vi "cleanRAWobj.vi"(8 "error in (no error)":errorcluster, 11 "raw dxf obj in":string) -> (0 "error out":errorcluster, 3 "dxfObject":T1, 5 "complete obj as 2Darray out":string[][](array[string]))   [LabVIEW 2016, in "Dxf.lvlib"]
uses:
  Dxf.lvlib
  typeDefs/singleDXFobject.ctl
  typeDefs/singleDXFvar.ctl
  <vilib>/Utility/error.llb/whitespace.ctl
  dxf typedef.lvlib
panel:
  out "raw obj cleaned":string
  # "Connector Pane"
  # "Locals"
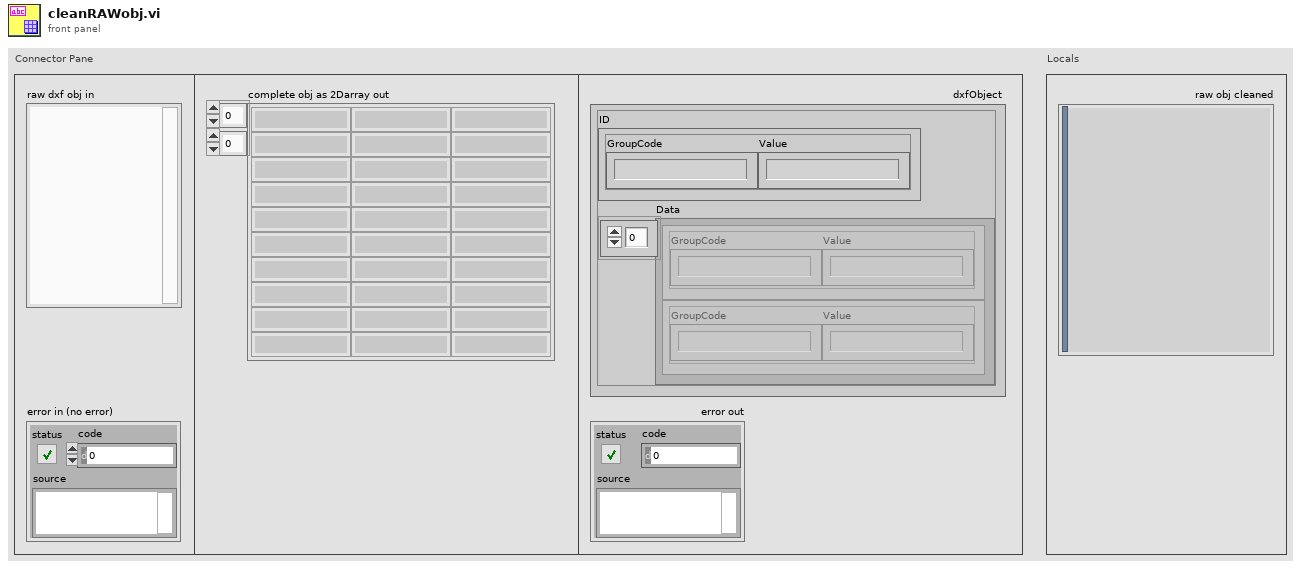
[diagram p1: front panel]
types:
  T1 = typedef "dxf typedef.lvlib/singleDXFobject.ctl" = cluster{"ID":T2, "Data":T2[]}
  T2 = typedef "dxf typedef.lvlib/singleDXFvar.ctl" = cluster{"GroupCode":string, "Value":string}
  T3 = typedef "whitespace.ctl" = u16
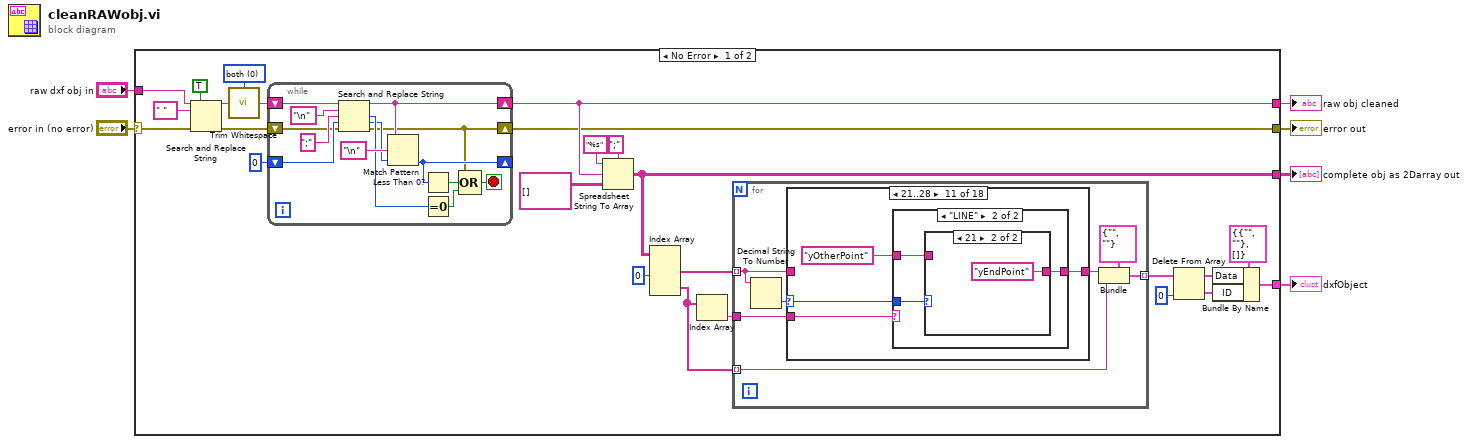
[diagram p0: block diagram]
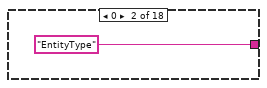
[diagram p3: hidden frame]
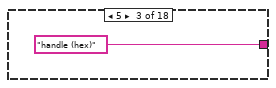
[diagram p4: hidden frame]
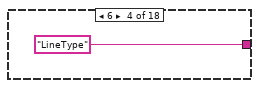
[diagram p5: hidden frame]
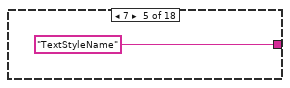
[diagram p6: hidden frame]
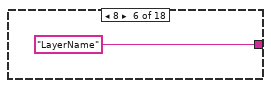
[diagram p7: hidden frame]
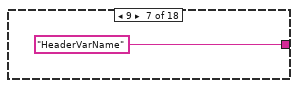
[diagram p8: hidden frame]
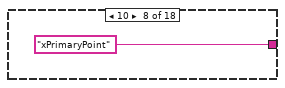
[diagram p9: hidden frame]
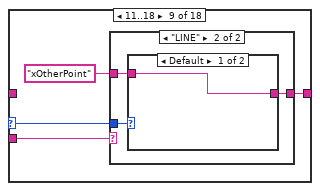
[diagram p10: hidden frame]
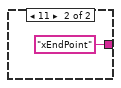
[diagram p12: hidden frame]
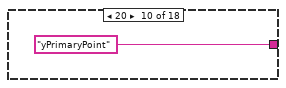
[diagram p13: hidden frame]
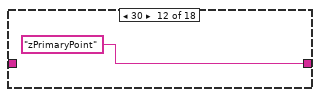
[diagram p16: hidden frame]
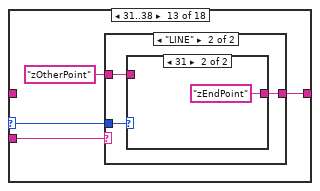
[diagram p17: hidden frame]
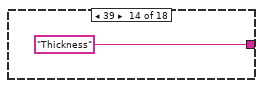
[diagram p20: hidden frame]
diagram:
  n1 = case shown="No Error" "error in (no error)" {
    selector: "error in (no error)" -> [w21 w122]
    tunnel: [w28 _] -> w6
    tunnel: [w17 _] -> w5
    tunnel: [w19 w122] -> w3
    tunnel: "raw dxf obj in" -> [w18 _]
    tunnel: [w12 _] -> w1
    frame No Error {
      w22 = T3 0 items=["both", "start of string", "end of string"] ("location (both)")
      n2 = Search and Replace String(replace all?=TRUE ("replace all? (F)"), input string=w18, search string=" ", error in=w21) -> (result string=w26:string, error out=w20:errorcluster)  [unwired: 4 in, 2 out]
      n3 = call <vilib>:"Trim Whitespace.vi"("string"=w26, "location (both)"=w22) -> ("trimmed string"=w23:string)
      n4 = while {
        shift-right: [w115] -> w28
        shift-left: w23 -> [w120]
        shift-right: [w111] -> _
        shift-left: 0 ("offset past match") -> [w116]
        shift-right: [w108] -> w19
        shift-left: w20 -> [w109]
        stop <- w114 stop-if-true
        n5 = Search and Replace String(input string=w120, search string="\n", replace string=";" ("replace string (\"\")"), offset=w116, error in=w109) -> (result string=w115:string, number of replacements=w113:i32, offset past replacement=w112:i32, error out=w108:errorcluster)  [unwired: 3 in]
        n6 = Match Pattern(string=w115, regular expression="\n" ("search string"), offset (0)=w112) -> (offset past match=w111:i32)  [unwired: 3 out]
        n7 = Less Than 0?(x=w111) -> (x < 0?=w110:bool)
        n8 = Equal To 0?(x=w113) -> (x = 0?=w121:bool)
        n9 = Compound Arithmetic op=OR(w108, w110, w121) -> (w114:bool)
      }
      n10 = Spreadsheet String To Array(delimiter (Tab)=";" ("search string"), format string="%s", spreadsheet string=w28, array type (2D Dbl)=string[][] []) -> (array=w17:string[][])
      n11 = Index Array(array=w17, index (col) #1=0 ("disabled index (col)")) -> (element #1=w15:string[], element #2=w14:string[])  [unwired: 3 in]
      n12 = Index Array(array=w14) -> (element=w13:string)  [unwired: 1 in]
      n13 = for {
        tunnel: w15 -> [w37] mode=indexing
        tunnel: w13 -> [w36]
        tunnel: w14 -> [w34] mode=indexing
        tunnel: [w33] -> w10 mode=indexing
        n14 = Decimal String To Number(string=w37) -> (number=w38:i32)  [unwired: 2 in, 1 out]
        n15 = case shown="21..28" w38 {
          selector: w38 -> [_ _ _ _ _ _ _ _ w47 _ w58 _ w69 _ w80 _ w97 _]
          tunnel: [w39 "EntityType" "handle (hex)" "LineType" "TextStyleName" "LayerName" "HeaderVarName" "xPrimaryPoint" w49 "yPrimaryPoint" w61 "zPrimaryPoint" w72 "Thickness" w82 "LinetypeScale" w99 "ColorNumber"] -> w35
          tunnel: w37 -> [w39 _ _ _ _ _ _ _ _ _ _ _ _ _ _ _ _ _]
          tunnel: w36 -> [_ _ _ _ _ _ _ _ w50 _ w59 _ w70 _ w83 _ w98 _]
          frame Default {
          }
          frame 0 {
          }
          frame 5 {
          }
          frame 6 {
          }
          frame 7 {
          }
          frame 8 {
          }
          frame 9 {
          }
          frame 10 {
          }
          frame 11..18 {
            n16 = case shown="\"LINE\"" w50 {
              tunnel: [w51 w53] -> w49
              tunnel: "xOtherPoint" -> [w51 w52]
              tunnel: w47 -> [_ w54]
              frame Default {
              }
              frame "LINE" {
                n17 = case shown="Default" w54 {
                  tunnel: [w55 "xEndPoint"] -> w53
                  tunnel: w52 -> [w55 _]
                  frame Default {
                  }
                  frame 11 {
                  }
                }
              }
            }
          }
          frame 20 {
          }
          frame 21..28 {
            n18 = case shown="\"LINE\"" w59 {
              tunnel: [w62 w65] -> w61
              tunnel: "yOtherPoint" -> [w62 w64]
              tunnel: w58 -> [_ w63]
              frame Default {
              }
              frame "LINE" {
                n19 = case shown="21" w63 {
                  tunnel: [w66 "yEndPoint"] -> w65
                  tunnel: w64 -> [w66 _]
                  frame Default {
                  }
                  frame 21 {
                  }
                }
              }
            }
          }
          frame 30 {
          }
          frame 31..38 {
            n20 = case shown="\"LINE\"" w70 {
              tunnel: [w73 w76] -> w72
              tunnel: "zOtherPoint" -> [w73 w75]
              tunnel: w69 -> [_ w74]
              frame Default {
              }
              frame "LINE" {
                n21 = case shown="31" w74 {
                  tunnel: [w77 "zEndPoint"] -> w76
                  tunnel: w75 -> [w77 _]
                  frame Default {
                  }
                  frame 31 {
                  }
                }
              }
            }
          }
          frame 39 {
          }
          frame 40..47 {
            n22 = case shown="\"ARC\"" w83 {
              tunnel: [w84 w86 w91] -> w82
              tunnel: "VarDoubleValue" -> [w84 w85 w90]
              tunnel: w80 -> [_ w87 w92]
              frame Default {
              }
              frame "CIRCLE" {
                n23 = case shown="40" w87 {
                  tunnel: [w88 "Radius"] -> w86
                  tunnel: w85 -> [w88 _]
                  frame Default {
                  }
                  frame 40 {
                  }
                }
              }
              frame "ARC" {
                n24 = case shown="40" w92 {
                  tunnel: [w93 "Radius"] -> w91
                  tunnel: w90 -> [w93 _]
                  frame Default {
                  }
                  frame 40 {
                  }
                }
              }
            }
          }
          frame 48 {
          }
          frame 50..58 {
            n25 = case shown="\"ARC\"" w98 {
              tunnel: [w100 w101] -> w99
              tunnel: "VarAngle (deg)" -> [w100 w102]
              tunnel: w97 -> [_ w103]
              frame Default {
              }
              frame "ARC" {
                n26 = case shown="50" w103 {
                  tunnel: w102 -> [w104 _ _]
                  tunnel: [w104 "StartAngle (deg)" "EndAngle (deg)"] -> w101
                  frame Default {
                  }
                  frame 50 {
                  }
                  frame 51 {
                  }
                }
              }
            }
          }
          frame 62 {
          }
        }
        n27 = Bundle(cluster=T2 {"GroupCode"="", "Value"=""}, "GroupCode"=w35, "Value"=w34) -> (w33:T2)
      }
      n28 = Delete From Array(array=w10, index=0) -> (deleted portion=w8:T2, array with subset deleted=w7:T2[])  [unwired: 1 in]
      n29 = Bundle By Name(cluster=T1 {"ID"={"GroupCode"="", "Value"=""}, "Data"=[]}, "Data"=w7, "ID"=w8) -> (w12:T1)
    }
    frame Error {
    }
  }
  "complete obj as 2Darray out" <- w5
  "raw obj cleaned" <- w6
  "error out" <- w3
  "dxfObject" <- w1
